vi "msgsBuilder_MasterMessage2.vi"(9 "Array":dbl[](array[numeric]), 10 "Position":cluster{"x":dbl, "y":dbl, "z":dbl}, 11 "PickingRoutine":i32) -> (3 "msg out":string)   [LabVIEW 2016]
uses:
  builds/UnicornMain/UnicornRIO1/ROS for LabVIEW/home/lvuser/natinst/bin/user.lib/ROS for LabVIEW Software/ROS/MessageBuilding/std_msgs/subs/i32Scalar.vi
  builds/UnicornMain/UnicornRIO1/ROS for LabVIEW/home/lvuser/natinst/bin/user.lib/ROS for LabVIEW Software/ROS/MessageBuilding/std_msgs/subs/float32Array.vi
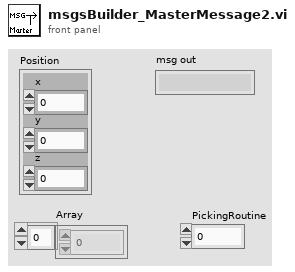
[diagram p1: front panel]
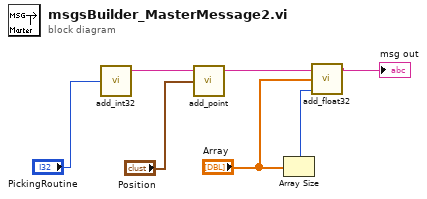
[diagram p0: block diagram]
diagram:
  n1 = call-poly "add_int32.vi"("Numeric"="PickingRoutine") -> ("msg out"=w1:string)  [unwired: 4 in]
  n2 = call "add_point.vi"("Point"="Position", "msg in"=w1) -> ("msg out"=w6:string)  [unwired: 3 in]
  n3 = Array Size(array="Array") -> (size(s)=w3:i32)
  n4 = call-poly "add_float32.vi"("Array Length"=w3, "Array"="Array", "msg in"=w6) -> ("msg out"=→"msg out":string)  [unwired: 2 in]
